vi "Static Write.vi"(8 "error in (no error)":errorcluster, 10 "Value":timestamp, 11 "Abs_Time in":refnum<class "Abs_Time.lvclass">) -> (0 "error out":errorcluster, 3 "Abs_Time out":refnum<class "Abs_Time.lvclass">)   [LabVIEW 2021, in "Abs_Time.lvclass"]
uses:
  Abs_Time.lvclass
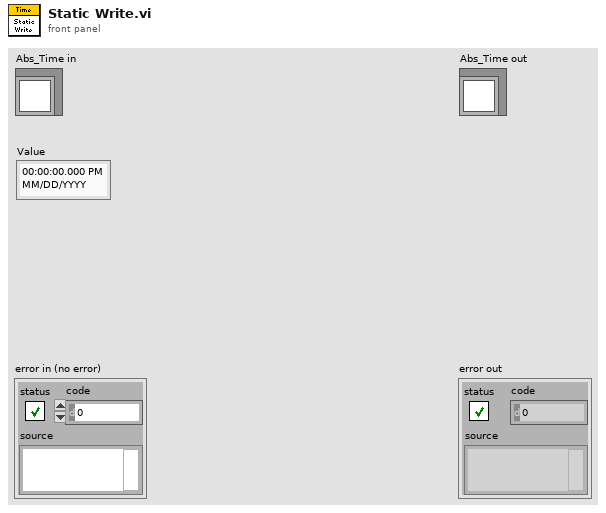
[diagram p1: front panel]
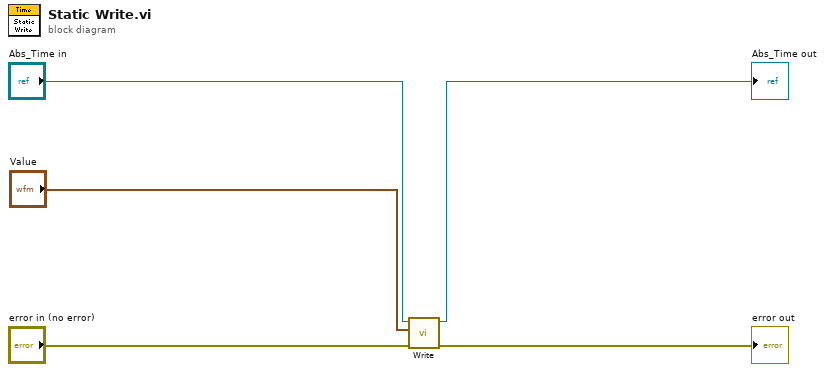
[diagram p0: block diagram]
diagram:
  n1 = call-dynamic "Write.vi"("error in (no error)"="error in (no error)", "Value"="Value", "Double Float.lvclass_340760 in"="Abs_Time in") -> ("error out"=→"error out":errorcluster, "Double Float.lvclass_340760 out"=→"Abs_Time out":refnum<class "Abs_Time.lvclass">)  [unwired: 7 in]
